vi "xiCam - Get1DImageData.vi"(7 "timeout":i32, 8 "error in (no error)":errorcluster, 9 "1DImageData In":u8[](array[numeric]), 11 "xiCam In":refnum<k24>) -> (0 "error out":errorcluster, 1 "1DImageData Out":u8[](array[numeric]), 3 "xiCam Out":refnum<k24>, 4 "Image Properites":T1)   [LabVIEW 2015]
doc: "This function acquires image and returns a preallocated byte array containing the Image data.\n\n<b>void GetImage(byte* ImageData, int timeout)</b>\nint timeout : Time interval required to wait for the image (in milliseconds)"
uses:
  Utils/xiImageManager/xiImageMng - State.ctl
  C:/GIT/Cameras3.x/Integrations/Labview/xiLib/xiLIB_32bit/xiLIB/xiCamLib/API/x86/xiApi.NET.dll
  xiLIB_32bit/xiLIB/xiCamLib/API/x86/xiApi.NET.dll
  Utils/xiImageManager/xiImageMng - Attributes.ctl
  PRM/IMG_FORMAT/IMG_DATA_FORMAT.ctl
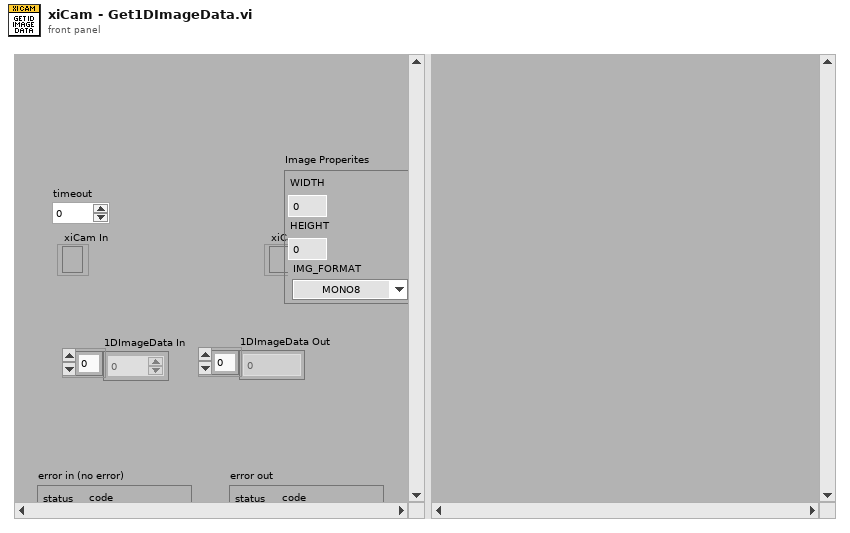
[diagram p1: front panel]
types:
  T1 = typedef "xiImageMng - Attributes.ctl" = cluster{"WIDTH":i32, "HEIGHT":i32, "IMG_FORMAT":T2}
  T2 = typedef "IMG_DATA_FORMAT.ctl" = enum16{"MONO8", "MONO16", "RGB24", "RGB32", "RGBPLANAR", "RAW8", "RAW16"}
  T3 = typedef "xiImageMng - State.ctl" = enum16{"Init", "GetProperties", "SetProperties"}
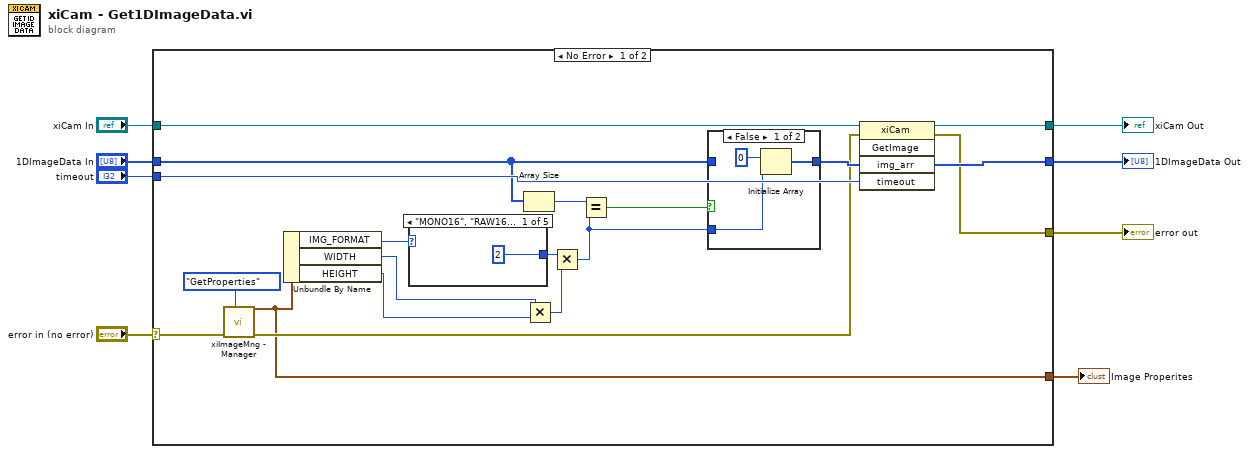
[diagram p0: block diagram]
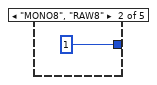
[diagram p2: hidden frame]
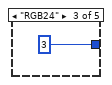
[diagram p3: hidden frame]
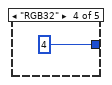
[diagram p4: hidden frame]
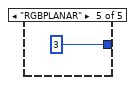
[diagram p5: hidden frame]
diagram:
  n1 = case shown="No Error" "error in (no error)" {
    selector: "error in (no error)" -> [w21 w37]
    tunnel: "xiCam In" -> [w27 w38]
    tunnel: [w26 w38] -> w6
    tunnel: [w23 w37] -> w5
    tunnel: "timeout" -> [w25 _]
    tunnel: [w24 _] -> w3
    tunnel: "1DImageData In" -> [w16 _]
    tunnel: [w13 _] -> w1
    frame No Error {
      n2 = call "xiImageMng - Manager.vi"("State"=xiImageMng_-_State."GetProperties", "error in (no error)"=w21) -> ("error out"=w14:errorcluster, "Properties Out"=w13:T1)  [unwired: 8 in]
      n3 = Unbundle By Name(w13) -> ("IMG_FORMAT"=w10:T2, "WIDTH"=w20:i32, "HEIGHT"=w19:i32)
      n4 = case shown="\"MONO16\", \"RAW16\"" w10 {
        tunnel: [2 ("x*y") 1 ("x*y") 3 ("x*y") 4 ("x*y") 3 ("x*y")] -> w9
        frame "MONO16", "RAW16" {
        }
        frame "MONO8", "RAW8" {
        }
        frame "RGB24" {
        }
        frame "RGB32" {
        }
        frame "RGBPLANAR" {
        }
      }
      n5 = Array Size(array=w16) -> (size(s)=w18:i32)
      n6 = Multiply(x=w20, y=w19) -> (x*y=w12:i32)
      n7 = Multiply(x=w9, y=w12) -> (x*y=w11:i32)
      n8 = Equal?(x=w18, y=w11) -> (x = y?=w17:bool)
      n9 = case shown="False" w17 {
        tunnel: w16 -> [_ w36]
        tunnel: [w33 w36] -> w15
        tunnel: w11 -> [w34 _]
        frame False {
          n10 = Initialize Array(u8 0, w34) -> (w33:u8[])
        }
        frame True {
        }
      }
      n11 = invoke class="xiCam" method="GetImage"(reference=w27, error in=w14, "img_arr"=w15, "timeout"=w25) -> (reference out=w26:refnum<k24>, error out=w23:errorcluster, "img_arr"=w24:u8[])  [unwired: 1 in, 2 out]
    }
    frame Error {
    }
  }
  "error out" <- w5
  "xiCam Out" <- w6
  "1DImageData Out" <- w3
  "Image Properites" <- w1
